vi "MC.DangwooOptron.GetResource.vi"(8 "error in (no error)":errorcluster, 11 "MC.DangwooOptron":refnum<class "MC.DangwooOptron.lvclass">) -> (0 "error out":errorcluster, 2 "Resource":T1, 3 "MC.DangwooOptron out":refnum<class "MC.DangwooOptron.lvclass">)   [LabVIEW 2017, in "MC.DangwooOptron.lvclass"]
doc: "JKI State Machine Objects (SMO) 1.0.0.5\nJKI - JKI\nCopyright (c) 2016, JKI"
uses:
  MC.DangwooOptron.lvclass
  Typedefs/Resource--Cluster.ctl
  MC.DangwooOptron.lvclass/MC.DangwooOptron.ctl
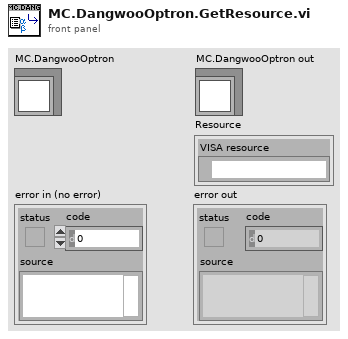
[diagram p1: front panel]
types:
  T1 = typedef "MC.DangwooOptron.lvclass/Resource--Cluster.ctl" = cluster{"VISA resource":refnum<visa-resource-name>}
  T2 = typedef "MC.DangwooOptron.lvclass/PrivateData--Ref.ctl" = refnum<data-value>
  T3 = typedef "MC.DangwooOptron.lvclass/PrivateData--Cluster.ctl" = cluster{"Resource":T1}
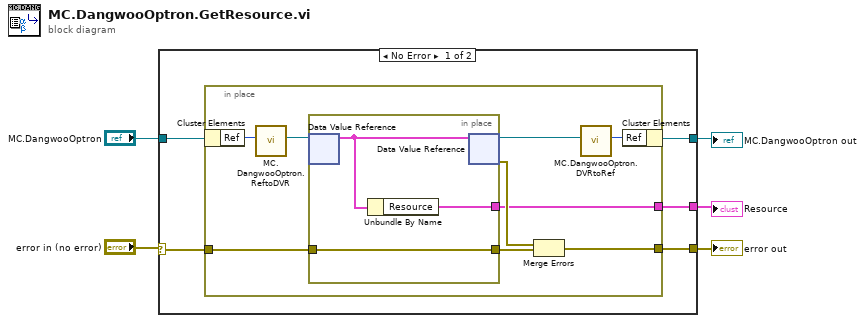
[diagram p0: block diagram]
diagram:
  n1 = case shown="No Error" "error in (no error)" {
    selector: "error in (no error)" -> [w8 w23]
    tunnel: [w10 w24] -> w5
    tunnel: "MC.DangwooOptron" -> [w9 w24]
    tunnel: [w7 w23] -> w2
    tunnel: [w6 _] -> w1
    frame No Error {
      n2 = in-place {
        in-place-border: w8 -> [w16]
        in-place-border: [w12] -> w7
        in-place-border: [w11] -> w6
        n3 = in-place-cluster #1(w9) -> ("Ref"=w19:u32)
        n4 = call "MC.DangwooOptron.ReftoDVR.vi"("Ref"=w19) -> ("Ref"=w18:T2)  [unwired: 10 in]
        n5 = in-place {
          in-place-border: w16 -> [w22]
          in-place-border: [w22] -> w14
          in-place-border: [w20] -> w11
          n6 = in-place-dvr #2(w18) -> (w21:T3)  [unwired: 1 out]
          n7 = Unbundle By Name(w21) -> ("Resource"=w20:T1)
          n8 = in-place-dvr #2(w21) -> (w15:T2, w13:errorcluster)
        }
        n9 = Merge Errors(w13, w14) -> (w12:errorcluster)
        n10 = call "MC.DangwooOptron.DVRtoRef.vi"("Ref"=w15) -> ("Ref"=w17:u32)  [unwired: 10 in]
        n11 = in-place-cluster #1("Ref"=w17) -> (w10:refnum<class "MC.DangwooOptron.lvclass">)
      }
    }
    frame Error {
    }
  }
  "error out" <- w2
  "MC.DangwooOptron out" <- w5
  "Resource" <- w1
